vi "Gui_SetupTiming.vi"(7 "Variant For Path":variant, 8 "error in (no error)":errorcluster, 11 "Variant":variant) -> (0 "error out":errorcluster caption="sortie d'erreur", 3 "Variant Output":variant)   [LabVIEW 2017]
uses:
  controls/SEQUENCE_Inputs.ctl
  controls/TRAPPING_Inputs.ctl
  controls/EXCIT_Inputs.ctl
  controls/DATA_Inputs.ctl
  controls/TIMING_Inputs.ctl
  controls/PROCESSING_Inputs.ctl
  controls/EXPERT_Inputs.ctl
  controls/DIGIT_5122_Inputs.ctl
  <instrlib>/niScope/Controls/niScope trigger source.ctl
  controls/HSDIO_6541_Inputs.ctl
  <instrlib>/niHSDIO/niHSDIO.llb/niHSDIO_ctl Trigger Source Values (Ring).ctl
  controls/SOFTWARE_Inputs.ctl
  controls/AO_6711_Inputs.ctl
  controls/AWG_5421_Inputs.ctl
  <instrlib>/niFgen/niFgen.llb/niFgen_ctl Trigger Source Values (Ring).ctl
  controls/XML_Inputs.ctl
panel:
  in  "EXPERT Inputs":T1={"DIGIT 5122 Inputs"={"Sample Rate"=9.0, "Resource Name"="Digitizer", "Channel Name"="0", "Trigger Source"="VAL_EXTERNAL", "Vertical Range"=10.0, "Trigger Level"=3.0}, "HSDIO 6541 Inputs"={"Resource Name"="SequencerHSDIO", "Clock Rate"=1000000.0, "Trigger Source"="PFI0"}, "SOFTWARE Inputs"={"Application Directory"=path "D:/S.O.F.T.S/LABVIEW/PIL", "Software Version"="1.0.0", "Data Path"=path "D:/PIRENEA/DATA", "XML Path"=path "D:/PIRENEA/DATA", "XML File Filter"="*.xml", "XML Saved Path"=path "D:/PIRENEA/DATA", "Excit Scripts Path"=path "D:/PIRENEA/EXCIT_SCRIPTS", "Excit Scripts File Filter"="*.txt", "Excit Waveforms Path"=path "D:/PIRENEA/EXCIT_WFMS", "Excit Waveforms File Filter"="*.bin", "Timing Scripts Path"=path "D:/PIRENEA/SEQUENCE_SCRIPTS", "Timing Scripts File Filter"="*.txt", "Timing Waveforms Path"=path "D:/PIRENEA/SEQUENCE_WFMS", "Timing Waveforms File Filter"="*.bin", "Trapping Waveforms Path"=path "D:/PIRENEA/TRAPPING_WFMS", "Trapping Waveforms File Filter"="*.bin"}, "AO 6711 Inputs"={"Physical Channels"="AnalogOutput/ao0:3", "Min Voltage"=-10.0, "Max Voltage"=10.0, "Trigger Source"="/AnalogOutput/PFI0", "Counter"="AnalogOutput/ctr0"}, "AWG 5421 Inputs"={"Resource Name"="WaveformGenerator", "Sample Rate"=20000000.0, "Trigger Type"=2, "Trigger Source"="PFI0", "Waveform Gain"=0.31, "Digital Filter ON"=TRUE}, "XML Inputs"={"Version Tag Name"="XML_Version", "Version String"="1.0"}} {"AWG 5421 Inputs"."Sample Rate" format="%.2p"; "AWG 5421 Inputs"."Trigger Type" items=["None", "Software Edge", "Digital Edge", "Digital Level"]; "AO 6711 Inputs"."Max Voltage" min=-10.0 max=10.0; "AO 6711 Inputs"."Min Voltage" min=-10.0 max=10.0; "HSDIO 6541 Inputs"."Clock Rate" format="%.2p"; "DIGIT 5122 Inputs"."Trigger Level" format="%.2f"; "DIGIT 5122 Inputs"."Vertical Range" format="%.2f"; "DIGIT 5122 Inputs"."Sample Rate" step=65535.0 format="%#_3p"}
  in  "SEQUENCE Inputs":T11={"TRAPPING Inputs"={"Number of Channels"=4, "Init Values"=[2.0, 5.0, 5.0, 2.0], "Opening Values"=[0.0, 0.0, 0.0, 0.0], "Trapping Values"=[2.0, 5.0, 5.0, 2.0], "Emptying Values"=[-5.0, -5.0, -5.0, -5.0], "Adiabatic ON"=FALSE, "Adiabatic Duration"=0, "Adiabatic Waveforms"=["Adiabatic_None_2_2_2000.bin", "Adiabatic_Ramp_5_0_2000.bin", "Adiabatic_DoubleRamp_5_0_2000.bin", "Adiabatic_RC_2_0_2000.bin"]}, "EXCIT Inputs"={"Number of Excitations"=1, "Script Text"="", "Table of Waveforms"=[]}, "DATA Inputs"={"Record Length"=8192, "Sample Rate"=4.0, "Data Type"=0, "Vertical Range"=0.0, "Acquisition Duration"=100000.0}, "TIMING Inputs"={"Number of Acquisitions "=1, "Number of Accumulations"=1, "Table of Waveforms"=[], "Script Text"=""}, "PROCESSING  Inputs"={"Reference Mass"=300.0939, "Cyclotron Freq"=255.727, "Magnetron Freq"=0.001}} {"PROCESSING  Inputs"."Magnetron Freq" format="%.5g"; "PROCESSING  Inputs"."Cyclotron Freq" format="%.5g"; "PROCESSING  Inputs"."Reference Mass" format="%.5g"; "TIMING Inputs"."Number of Accumulations" min=0 max=50 step=1; "TIMING Inputs"."Number of Acquisitions" min=1 max=10 step=1; "DATA Inputs"."Vertical Range" items=["0.2"=0.2, "0.4"=0.4, "1"=1.0, "2"=2.0, "4"=4.0, "10"=10.0]; "DATA Inputs"."Data Type" items=["I16", "DBL"]; "DATA Inputs"."Sample Rate" items=["1 MHz"=1000000.0, "2 MHz"=2000000.0, "5 MHz"=5000000.0, "10 MHz"=10000000.0, "20 MHz"=20000000.0, "25 MHz"=25000000.0, "50 MHz"=50000000.0, "100 MHz"=100000000.0]; "EXCIT Inputs"."Number of Excitations" min=1 max=10; "TRAPPING Inputs"."Trapping Values" min=-10.0 max=10.0; "TRAPPING Inputs"."Init Values" min=-10.0 max=10.0; "TRAPPING Inputs"."Emptying Values" min=-10.0 max=10.0; "TRAPPING Inputs"."Opening Values" min=-10.0 max=10.0}
  out "Number Of Excitations":i16=1 min=1 max=10 step=1
  in  "Number Of Accumulations":i16=1 min=0 max=50 step=1
  out "Number Of Acquisitions":i16=1 min=1 max=10 step=1
  in  "Table of Scripts":string[](array[string])=["script PireneaEject2sGas2sExcitAcq8s\n   wait until scriptTrigger0 \n   wait 949940\n   generate AutLaserOn\n   wait 49000\n   generate AutLaserOnFilterOff\n   wait 1000\n   wait 600\n   generate AutLaserOnFilterOffTrapStart\n   wait 300\n   generate AutLaserOnFilterOffTrapStop\n   wait 2000\n   generate AutLaserOnFilterOn\n   wait 47100\n   generate AutLaserOff\n   wait 1950000\n   generate Excit\n   wait 50000\n   generate Gas1On\n   wait 150000\n   generate GasOff\n   wait 5800000\n   generate ExcitAcq\n   wait 1000000\n   generate FilterOff\n   wait 1000\n   generate FilterOffEmptyingStart\n   wait 1000000\n   generate FilterOffEmptyingStop\n   wait 2000\n   generate Zeros\nend script", "script PireneaExcitAcq1min\n   wait until scriptTrigger0 \n   wait 949940\n   generate AutLaserOn\n   wait 49000\n   generate AutLaserOnFilterOff\n   wait 1000\n   wait 600\n   generate AutLaserOnFilterOffTrapStart\n   wait 300\n   generate AutLaserOnFilterOffTrapStop\n   wait 2000\n   generate AutLaserOnFilterOn\n   wait 47100\n   generate AutLaserOff\n   wait 59950000\n   generate ExcitAcq\n   wait 10000000\n   generate FilterOff\n   wait 2000\n   generate FilterOffEmptyingStart\n   wait 1000000\n   generate FilterOffEmptyingStop\n   wait 2000\n   generate Zeros\nend script", "script PireneaExcitAcq4s\n   wait until scriptTrigger0 \n   wait 949940\n   generate AutLaserOn\n   wait 49000\n   generate AutLaserOnFilterOff\n   wait 1000\n   wait 600\n   generate AutLaserOnFilterOffTrapStart\n   wait 300\n   generate AutLaserOnFilterOffTrapStop\n   wait 2000\n   generate AutLaserOnFilterOn\n   wait 47100\n   generate AutLaserOff\n   wait 3950000\n   generate ExcitAcq\n   wait 1000000\n   generate FilterOff\n   wait 1000\n   generate FilterOffEmptyingStart\n   wait 1000000\n   generate FilterOffEmptyingStop\n   wait 2000\n   generate Zeros\nend script", "script PireneaExcitAcq5sEmptyingExcitAcq7s\n   wait until scriptTrigger0 \n   wait 949940\n   generate AutLaserOn\n   wait 49000\n   generate AutLaserOnFilterOff\n   wait 1000\n   wait 600\n   generate AutLaserOnFilterOffTrapStart\n   wait 300\n   generate AutLaserOnFilterOffTrapStop\n   wait 2000\n   generate AutLaserOnFilterOn\n   wait 47100\n   generate AutLaserOff\n   wait 4950000\n   generate ExcitAcq\n   wait 1000000\n   generate FilterOff\n   wait 1000\n   generate FilterOffEmptyingStart\n   wait 1000000\n   generate FilterOffEmptyingStop\n   wait 2000\n   generate ExcitAcq\n   wait 1000000\n   generate Zeros\nend script", "script PireneaFree4sExcitAcq5s\n   wait until scriptTrigger0 \n   wait 949940\n   generate AutLaserOn\n   wait 49000\n   generate AutLaserOnFilterOff\n   wait 1000\n   wait 600\n   generate AutLaserOnFilterOffTrapStart\n   wait 300\n   generate AutLaserOnFilterOffTrapStop\n   wait 2000\n   generate AutLaserOnFilterOn\n   wait 47100\n   generate AutLaserOff\n   wait 3950000\n   generate Acq\n   wait 1000000\n   generate ExcitAcq\n   wait 1000000\n   generate FilterOff\n   wait 1000\n   generate FilterOffEmptyingStart\n   wait 1000000\n   generate FilterOffEmptyingStop\n   wait 2000\n   generate Zeros\nend script", "script PireneaFree5s\n   wait until scriptTrigger0 \n   wait 949940\n   generate AutLaserOn\n   wait 49000\n   generate AutLaserOnFilterOff\n   wait 1000\n   wait 600\n   generate AutLaserOnFilterOffTrapStart\n   wait 300\n   generate AutLaserOnFilterOffTrapStop\n   wait 2000\n   generate AutLaserOnFilterOn\n   wait 47100\n   generate AutLaserOff\n   wait 4950000\n   generate Acq\n   wait 1000000\n   generate FilterOff\n   wait 1000\n   generate FilterOffEmptyingStart\n   wait 1000000\n   generate FilterOffEmptyingStop\n   wait 2000\n   generate Zeros\nend script", "script PireneaGas2sExcitAcq8s\n   wait until scriptTrigger0 \n   wait 949940\n   generate AutLaserOn\n   wait 49000\n   generate AutLaserOnFilterOff\n   wait 1000\n   wait 600\n   generate AutLaserOnFilterOffTrapStart\n   wait 300\n   generate AutLaserOnFilterOffTrapStop\n   wait 2000\n   generate AutLaserOnFilterOn\n   wait 47100\n   generate AutLaserOff\n   wait 1950000\n   generate Gas1On\n   wait 150000\n   generate GasOff\n   wait 5850000\n   generate ExcitAcq\n   wait 1000000\n   generate FilterOff\n   wait 1000\n   generate FilterOffEmptyingStart\n   wait 1000000\n   generate FilterOffEmptyingStop\n   wait 2000\n   generate Zeros\nend script", "script ZAdiabatic1sduring200msExcitAcq4s\n   wait until scriptTrigger0 \n   wait 949940\n   generate AutLaserOn\n   wait 49000\n   generate AutLaserOnFilterOff\n   wait 1000\n   wait 600\n   generate AutLaserOnFilterOffTrapStart\n   wait 300\n   generate AutLaserOnFilterOffTrapStop\n   wait 2000\n   generate AutLaserOnFilterOn\n   wait 47100\n   generate AutLaserOff\n   wait 950000\n   repeat 2000\n      generate Adiabatic10FilterOff\n      wait 90\n   end repeat\n   wait 2800000\n   generate ExcitAcq\n   wait 1000000\n   generate FilterOff\n   wait 1000\n   generate FilterOffEmptyingStart\n   wait 1000000\n   generate FilterOffEmptyingStop\n   wait 2000\n   generate Zeros\nend script"]
  in  "OK":bool
  in  "List of Scripts":i32[](listbox)
  # "GO_out"
  # "Gout"
  # "GI_in"
  # "Gin"
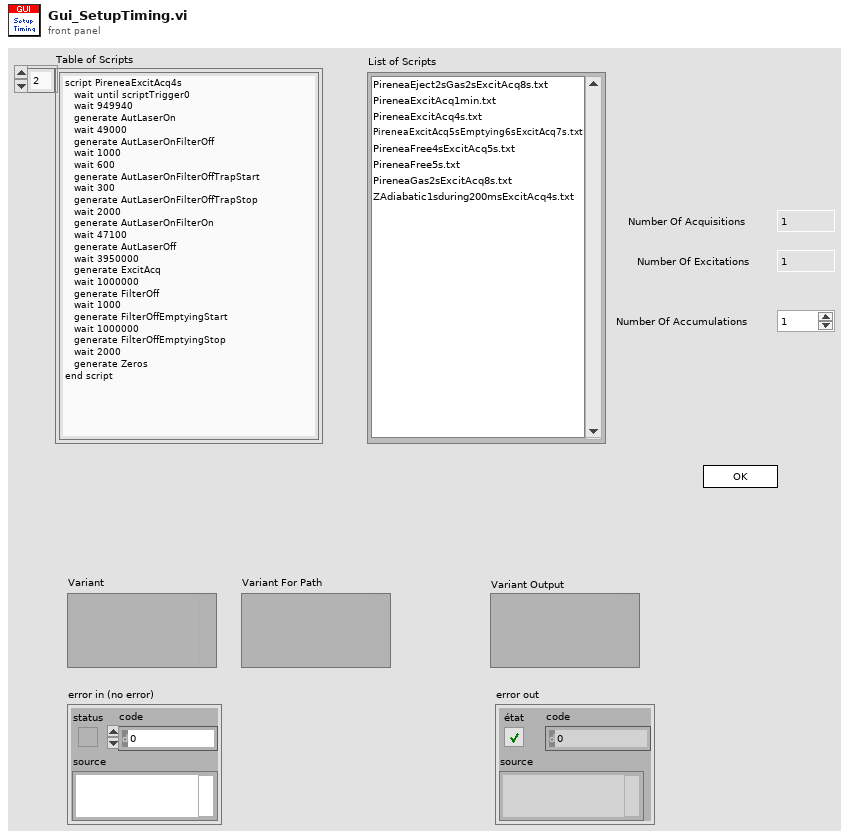
[diagram p1: front panel]
types:
  T1 = typedef "EXPERT_Inputs.ctl" = cluster{"DIGIT 5122 Inputs":T2, "HSDIO 6541 Inputs":T4, "SOFTWARE Inputs":T6, "AO 6711 Inputs":T7, "AWG 5421 Inputs":T8, "XML Inputs":T10}
  T2 = typedef "DIGIT_5122_Inputs.ctl" = cluster{"Sample Rate":dbl, "Resource Name":refnum<k15>, "Channel Name":string, "Trigger Source":T3, "Vertical Range":dbl, "Trigger Level":dbl}
  T3 = typedef "niScope trigger source.ctl" = string
  T4 = typedef "HSDIO_6541_Inputs.ctl" = cluster{"Resource Name":refnum<k15>, "Clock Rate":dbl, "Trigger Source":T5}
  T5 = typedef "niHSDIO_ctl Trigger Source Values (Ring).ctl" = string
  T6 = typedef "SOFTWARE_Inputs.ctl" = cluster{"Application Directory":path, "Software Version":string, "Data Path":path, "XML Path":path, "XML File Filter":string, "XML Saved Path":path, "Excit Scripts Path":path, "Excit Scripts File Filter":string, "Excit Waveforms Path":path, "Excit Waveforms File Filter":string, "Timing Scripts Path":path, "Timing Scripts File Filter":string, "Timing Waveforms Path":path, "Timing Waveforms File Filter":string, "Trapping Waveforms Path":path, "Trapping Waveforms File Filter":string}
  T7 = typedef "AO_6711_Inputs.ctl" = cluster{"Physical Channels":tag, "Min Voltage":dbl, "Max Voltage":dbl, "Trigger Source":tag, "Counter":tag}
  T8 = typedef "AWG_5421_Inputs.ctl" = cluster{"Resource Name":refnum<k15>, "Sample Rate":dbl, "Trigger Type":u16, "Trigger Source":T9, "Waveform Gain":dbl, "Digital Filter ON":bool}
  T9 = typedef "niFgen_ctl Trigger Source Values (Ring).ctl" = string
  T10 = typedef "XML_Inputs.ctl" = cluster{"Version Tag Name":string, "Version String":string}
  T11 = typedef "SEQUENCE_Inputs.ctl" = cluster{"TRAPPING Inputs":T12, "EXCIT Inputs":T13, "DATA Inputs":T14, "TIMING Inputs":T15, "PROCESSING  Inputs":T16}
  T12 = typedef "TRAPPING_Inputs.ctl" = cluster{"Number of Channels":i32, "Init Values":dbl[], "Opening Values":dbl[], "Trapping Values":dbl[], "Emptying Values":dbl[], "Adiabatic ON":bool, "Adiabatic Duration":i32, "Adiabatic Waveforms":string[]}
  T13 = typedef "EXCIT_Inputs.ctl" = cluster{"Number of Excitations":i32, "Script Text":string, "Table of Waveforms":string[]}
  T14 = typedef "DATA_Inputs.ctl" = cluster{"Record Length":i32, "Sample Rate":dbl, "Data Type":u8, "Vertical Range":dbl, "Acquisition Duration":dbl}
  T15 = typedef "TIMING_Inputs.ctl" = cluster{"Number of Acquisitions ":i16, "Number of Accumulations":i16, "Table of Waveforms":string[], "Script Text":string}
  T16 = typedef "PROCESSING_Inputs.ctl" = cluster{"Reference Mass":dbl, "Cyclotron Freq":dbl, "Magnetron Freq":dbl}
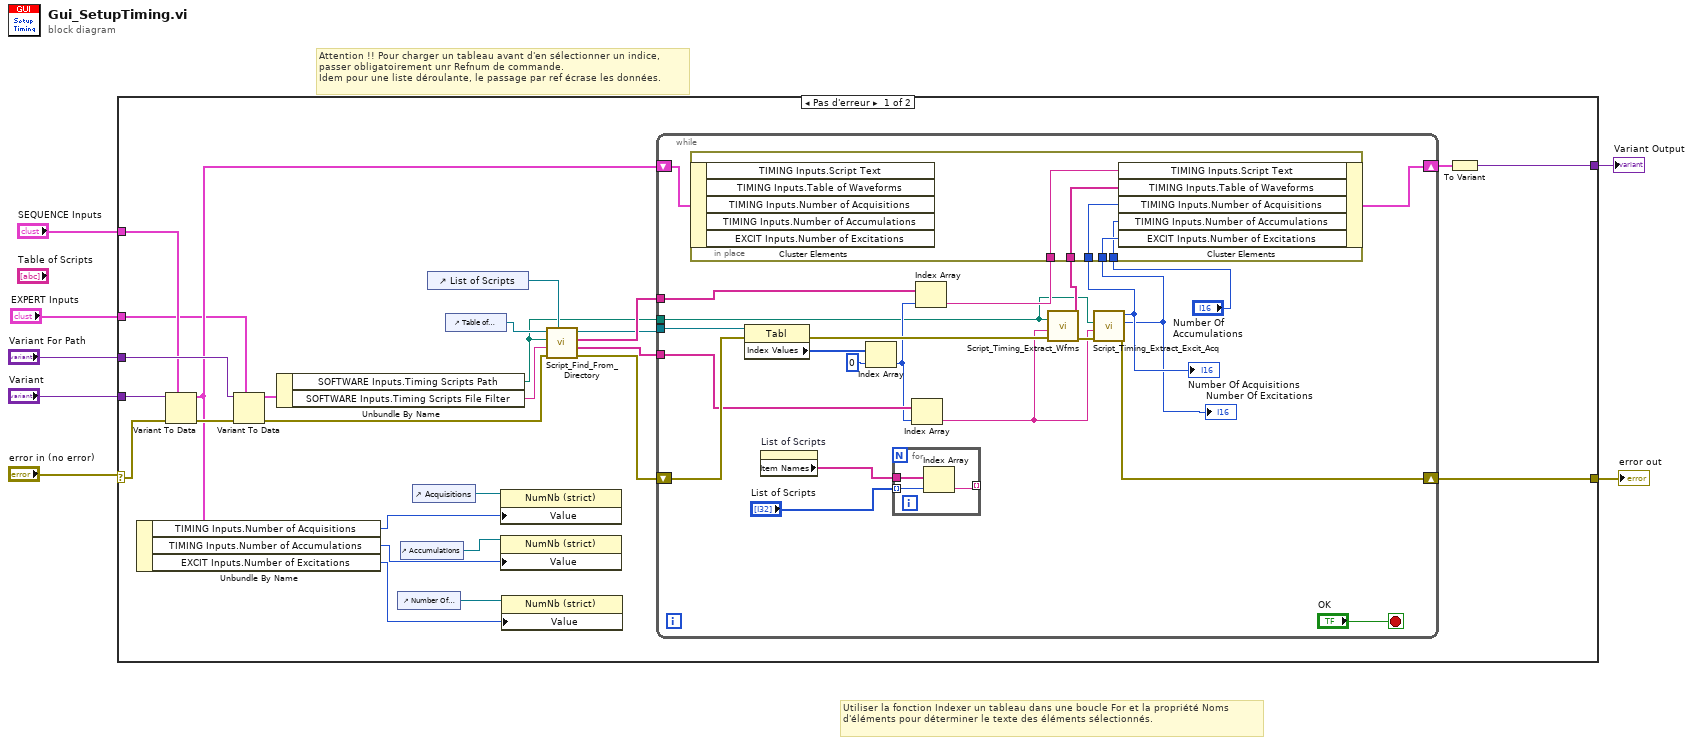
[diagram p0: block diagram]
diagram:
  # "Attention !! Pour charger un tableau avant d'en sélectionner un indice,\npasser obligatoirement unr Refnum de commande.\nIdem pour une liste déroulante, le passage par ref écrase les données."
  # "Utiliser la fonction Indexer un tableau dans une boucle For et la propriété Noms d'éléments pour déterminer le texte des éléments sélectionnés."
  n1 = case shown="Pas d'erreur" "error in (no error)" {
    selector: "error in (no error)" -> [w24 w65]
    tunnel: "Variant" -> [w27 w64]
    tunnel: [w26 w65] -> w5
    tunnel: [w25 w64] -> w4
    tunnel: "Variant For Path" -> [w21 _]
    tunnel: "SEQUENCE Inputs" -> [w9 _]
    tunnel: "EXPERT Inputs" -> [w8 _]
    frame No Error {
      n2 = Variant To Data(error in=w24, type=w9, Variant=w27) -> (data=w16:T11, error out=w23:errorcluster)
      n3 = Unbundle By Name(w16) -> ("TIMING Inputs.Number of Acquisitions"=w14:i16, "TIMING Inputs.Number of Accumulations"=w13:i16, "EXCIT Inputs.Number of Excitations"=w11:i32)
      n4 = Variant To Data(error in=w23, type=w8, Variant=w21) -> (data=w20:T1, error out=w22:errorcluster)
      n5 = Unbundle By Name(w20) -> ("SOFTWARE Inputs.Timing Scripts Path"=w18:path, "SOFTWARE Inputs.Timing Scripts File Filter"=w19:string)
      n6 = control-ref of="Number Of Excitations"() -> (w10:refnum<vi>)
      n7 = control-ref of="Accumulations"() -> (w12:refnum<vi>)
      n8 = control-ref of="Acquisitions"() -> (w15:refnum<vi>)
      n9 = control-ref of="List of Scripts"() -> (w31:refnum<vi>)
      n10 = control-ref of="Table of Scripts"() -> (w32:refnum<vi>)
      n11 = property class="NumNb (strict)"(reference=w15, "Value"=w14) -> ()  [unwired: 1 in, 2 out]
      n12 = property class="NumNb (strict)"(reference=w12, "Value"=w13) -> ()  [unwired: 1 in, 2 out]
      n13 = property class="NumNb (strict)"(reference=w10, "Value"=w11) -> ()  [unwired: 1 in, 2 out]
      n14 = call "Script_Find_From_Directory.vi"("Refnum LstDér"=w31, "error in (no error)"=w22, "Timing Scripts File Filter"=w19, "Timing Scripts Path"=w18, "Refnum Tabl"=w32) -> ("error out"=w28:errorcluster, "List of Scripts"=w29:string[], "Table of Scripts"=w33:string[], "Refnum Tabl Out"=w30:refnum<vi>)  [unwired: 2 in, 1 out]
      n15 = while {
        shift-right: [w42] -> w17
        shift-left: w16 -> [w44]
        tunnel: w33 -> [w52]
        tunnel: w30 -> [w51]
        tunnel: w29 -> [w48]
        shift-right: [w39] -> w26
        shift-left: w28 -> [w50]
        tunnel: w18 -> [w37]
        stop <- "OK" stop-if-true
        n16 = property on="Nœud de propriété" class="Tabl"(reference=w51, error in=w50) -> (error out=w49:errorcluster, "Index Values"=w54:u32[])  [unwired: 1 out]
        n17 = property on="List of Scripts" class="LstDér (strict)"() -> ("Item Names"=w46:string[])  [unwired: 2 in, 2 out]
        n18 = Index Array(array=w54, index=0 ("indice")) -> (element=w47:u32)
        n19 = for {
          tunnel: [w63] -> _ mode=indexing
          tunnel: w46 -> [w62]
          tunnel: "List of Scripts" -> [w61] mode=indexing
          n20 = Index Array(array=w62, index=w61) -> (element=w63:string)
        }
        n21 = Index Array(array=w48, index=w47) -> (element=w38:string)
        n22 = Index Array(array=w52, index=w47) -> (element=w41:string)
        n23 = call "Script_Timing_Extract_Wfms.vi"("error in (no error)"=w49, "Script File"=w38, "Script Path"=w37) -> ("error out"=w40:errorcluster, "Table of Waveforms"=w43:string[])  [unwired: 7 in]
        n24 = call "Script_Timing_Extract_Excit_Acq.vi"("error in (no error)"=w40, "Script File"=w38, "Script Path"=w37) -> ("error out"=w39:errorcluster, "Number of Excits"=w34:i16, "Number of Acqs"=w36:i16)  [unwired: 6 in]
        "Number Of Acquisitions" <- w36
        "Number Of Excitations" <- w34
        n25 = in-place {
          in-place-border: w41 -> [w60]
          in-place-border: w43 -> [w59]
          in-place-border: w36 -> [w58]
          in-place-border: w34 -> [w57]
          in-place-border: "Number Of Accumulations" -> [w56]
          n26 = in-place-cluster #1(w44) -> ()  [unwired: 5 out]
          n27 = in-place-cluster #1("TIMING Inputs.Script Text"=w60, "TIMING Inputs.Table of Waveforms"=w59, "TIMING Inputs.Number of Acquisitions"=w58, "TIMING Inputs.Number of Accumulations"=w56, "EXCIT Inputs.Number of Excitations"=w57) -> (w42:T11)
        }
      }
      n28 = To Variant(anything=w17) -> (Variant=w25:variant)
    }
    frame Error {
    }
  }
  "error out" <- w5
  "Variant Output" <- w4
